vi "ResonanceAnalyzer.vi"() -> ()   [LabVIEW 2015]
uses:
  <vilib>/imath/engines/lvmath2/RunTimeEngine/Managers/WorkSpace/UID Generator.vi
  <vilib>/imath/engines/lvmath2/RunTimeEngine/RangeToken/NIMS_Range.vi
  <instcachedir>/0/NIMS_Range_D919CC09935940E88F755EC1C6F49AC1.lvgen/NIMS_Range_D919CC09935940E88F755EC1C6F49AC1_000.vi
  <vilib>/imath/engines/lvmath2/RunTimeEngine/RunTimeType/NIMS_RunTimeType_From StrictType (excl LVString).vi
  <instcachedir>/0/NIMS_RunTimeType_From StrictType (excl LVString)_EB1C38A9BC5048DA9ABDA8F781E54D21.lvgen/NIMS_RunTimeType_From StrictType (excl LVString)_EB1C38A9BC5048DA9ABDA8F781E54D21_000.vi
  <vilib>/imathl/engines/lvmath/Functions/Error Handling/Create Error.vi
  <vilib>/imath/engines/lvmath2/RunTimeEngine/LocalVariableDefStatement/MC_LocalVariableDefStatement_Display.vi
  <vilib>/imath/engines/lvmath2/RunTimeEngine/ArithmeticOperatorToken/NIMS_ArithmeticOperator_minus.vi
  <instcachedir>/0/NIMS_ArithmeticOperator_minus_8228ED1EA52B4CB8A68367813E4B0C9D.lvgen/NIMS_ArithmeticOperator_minus_8228ED1EA52B4CB8A68367813E4B0C9D_003.vi
  <vilib>/imath/engines/lvmath2/RunTimeEngine/BuiltInFunctions/randnormal/NIMS_randnormal(1,I32).vi
  <vilib>/imath/engines/lvmath2/RunTimeEngine/ErrorHandling/NIMS_Error From Error Code.vi
  <vilib>/imath/engines/lvmath2/RunTimeEngine/ArithmeticOperatorToken/NIMS_ArithmeticOperator_plus.vi
  <instcachedir>/0/NIMS_ArithmeticOperator_plus_A4F2756F5ADB4A0090E0DBD7C10701C8.lvgen/NIMS_ArithmeticOperator_plus_A4F2756F5ADB4A0090E0DBD7C10701C8_000.vi
  <vilib>/imath/engines/lvmath2/RunTimeEngine/Managers/SymbolTable/Clear UID.vi
  <vilib>/imath/engines/lvmath2/RunTimeEngine/NodeEndStatement/NIMS_NodeEndStatement_Output.vi
  <instcachedir>/0/NIMS_NodeEndStatement_Output_53EC0D466D134D7ABD903AC30B43404B.lvgen/NIMS_NodeEndStatement_Output_53EC0D466D134D7ABD903AC30B43404B_000.vi
  <instcachedir>/0/NIMS_NodeEndStatement_Output_53EC0D466D134D7ABD903AC30B43404B.lvgen/NIMS_NodeEndStatement_Output_53EC0D466D134D7ABD903AC30B43404B_005.vi
  <vilib>/imath/engines/lvmath2/RunTimeEngine/ErrorHandling/NIMS_Finalize Error.vi
  <vilib>/imath/engines/lvmath2/RunTimeEngine/Managers/SymbolTable/NIMS_WorkSpace.lvlib
panel:
  out "Resonance Curve":cluster{"all rows":dbl[], "gaus":dbl[]}[](graph)=[{"all rows"=[400.0, 405.0, 410.0, 415.0, 420.0, 425.0, 430.0, 435.0, 440.0, 445.0, 450.0, 455.0, 460.0, 465.0, 470.0, 475.0, 480.0, 485.0, 490.0, 495.0, 500.0, 505.0, 510.0, 515.0, 520.0, 525.0, 530.0, 535.0, 540.0, 545.0, 550.0, 555.0, 560.0, 565.0, 570.0, 575.0, 580.0, 585.0, 590.0, 595.0, 600.0, 605.0, 610.0, 615.0, 620.0, 625.0, 630.0, 635.0, 640.0, 645.0, 650.0, 655.0, 660.0, 665.0, 670.0, 675.0, 680.0, 685.0, 690.0, 695.0, 700.0, 705.0, 710.0, 715.0, 720.0, 725.0, 730.0, 735.0, 740.0, 745.0, 750.0, 755.0, 760.0, 765.0, 770.0, 775.0, 780.0, 785.0, 790.0, 795.0, 800.0], "gaus"=[0.11351255241604037, 0.10414222503354348, 0.14444483533821953, 0.12748302072615827, 0.14497389221892898, 0.14384673103899848, 0.13374578408031648, 0.14179280076944742, 0.17330958944267544, 0.15907169164132778, 0.16753655176934548, 0.16514207171692954, 0.17190989932736572, 0.19691614978271704, 0.20190504370869367, 0.19441310786291455, 0.2133039056485444, 0.22477415941804885, 0.23020971646198585, 0.24797121378470008, 0.2536933279412255, 0.2773465910547763, 0.301521430656102, 0.30956997750864884, 0.33249213036731134, 0.34901602097743123, 0.39769074122820985, 0.41031887916188703, 0.41035673261766525, 0.4711874530017596, 0.48766721146953573, 0.5492859462216138, 0.5898183790247801, 0.6438836611617386, 0.7018972947086338, 0.7573592265847696, 0.8210938003460564, 0.8853988418295023, 0.9371620585856762, 0.9801248705682459, 0.9925356919276602, 0.9826137332493343, 0.9416889179435013, 0.9038575366906659, 0.8387554089811039, 0.7514021523756544, 0.7110991566651323, 0.6551377055862742, 0.6094819615126883, 0.5538177650246402, 0.5319943007321655, 0.48910912426227615, 0.4664119707496909, 0.44299884166073034, 0.40749275213784797, 0.38106205184860775, 0.3556589604478616, 0.3525103630210351, 0.3440871075427643, 0.31533845119817244, 0.29976668536036305, 0.2783162631954814, 0.2906476775521945, 0.2780539999902984, 0.26105862787721157, 0.255426074204126, 0.24557287287082505, 0.23745403917037838, 0.2423146884104632, 0.23349863360954015, 0.2027924510768934, 0.2039658188408361, 0.19926647781431656, 0.19642032188296885, 0.19371971901273244, 0.1916702535490835, 0.18835962796664552, 0.17745845067880478, 0.17841560928600508, 0.171532214028235, 0.15443785512252695]}, {"all rows"=[400.0, 405.0, 410.0, 415.0, 420.0, 425.0, 430.0, 435.0, 440.0, 445.0, 450.0, 455.0, 460.0, 465.0, 470.0, 475.0, 480.0, 485.0, 490.0, 495.0, 500.0, 505.0, 510.0, 515.0, 520.0, 525.0, 530.0, 535.0, 540.0, 545.0, 550.0, 555.0, 560.0, 565.0, 570.0, 575.0, 580.0, 585.0, 590.0, 595.0, 600.0, 605.0, 610.0, 615.0, 620.0, 625.0, 630.0, 635.0, 640.0, 645.0, 650.0, 655.0, 660.0, 665.0, 670.0, 675.0, 680.0, 685.0, 690.0, 695.0, 700.0, 705.0, 710.0, 715.0, 720.0, 725.0, 730.0, 735.0, 740.0, 745.0, 750.0, 755.0, 760.0, 765.0, 770.0, 775.0, 780.0, 785.0, 790.0, 795.0, 800.0], "gaus"=[0.11892435654300736, 0.12282734325640836, 0.12692064160827352, 0.1312191490068874, 0.13573931751779073, 0.14049935888608772, 0.14551948218171426, 0.15082217013157131, 0.15643250148251903, 0.16237852831753594, 0.1686917191977432, 0.17540748141751927, 0.18256577865249124, 0.1902118639900121, 0.19839715292579332, 0.20718026658252003, 0.21662828236911227, 0.2268182377606916, 0.23783894298854777, 0.24979317016415276, 0.2628002993015277, 0.2769995145893434, 0.2925536541534718, 0.30965381719781526, 0.3285248112128024, 0.3494314541621426, 0.3726855845009083, 0.398653284759308, 0.4277611217393421, 0.46049883371853045, 0.4974132905863116, 0.5390837703827893, 0.5860602321846007, 0.6387328739972306, 0.6970835970975545, 0.7602583531668472, 0.8259306283577391, 0.889583744570278, 0.9442088756583177, 0.9813204872080571, 0.9938278398123565, 0.9794874661552115, 0.942116222283669, 0.8894089891945062, 0.8294446788572712, 0.7684099929054267, 0.71009198407197, 0.6563567849513765, 0.6078379714990343, 0.5644878254485798, 0.5259323812265361, 0.4916737817486462, 0.461195544276965, 0.4340121392138449, 0.40968870161218524, 0.38784564078411693, 0.36815616430643266, 0.3503408990520392, 0.3341617018584087, 0.3194156449035439, 0.3059295890974517, 0.29355547319307834, 0.28216631097381767, 0.271652830925331, 0.26192067362005517, 0.2528880613855749, 0.2444838622430286, 0.23664598032865905, 0.22932001551601336, 0.22245814461604568, 0.21601818494044386, 0.20996280811029483, 0.20425887787418834, 0.19887689052195087, 0.19379050040813722, 0.18897611628788566, 0.18441255675214577, 0.18008075514383087, 0.17596350603541955, 0.17204524672877594, 0.1683118683615231]}]
  out "Results":T1={"Amplitude"=0.9938486787549025, "Q"=9.964741129222524, "Center Frequency"=599.8050675226251}
  in  "?":enum32{"Simulation", "Experiment"}(tab)
  in  "Input Parameters":T2={"Q"=10.0, "End Frequency"=800.0, "df"=5.0, "Noise Level"=0.01, "Center Frequency"=600.0, "Start Frequency"=400.0}
  in  "file path (dialog if empty)":path
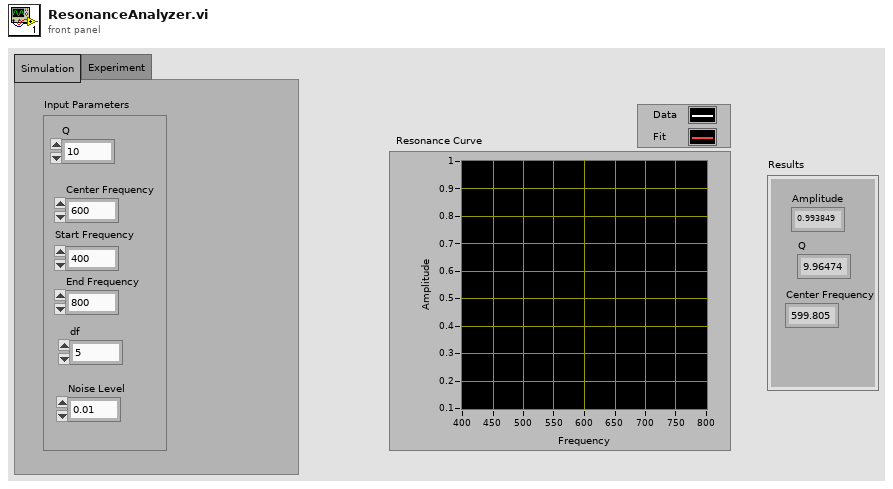
[diagram p1: front panel]
types:
  T1 = cluster{"Amplitude":dbl, "Q":dbl, "Center Frequency":dbl}
  T2 = cluster{"Q":dbl, "End Frequency":dbl, "df":dbl, "Noise Level":dbl, "Center Frequency":dbl, "Start Frequency":dbl}
  T3 = cluster{"Array[0]":dbl, "Array[1]":dbl, "Array[2]":dbl, "Array[3]":dbl, "Array[4]":dbl, "Array[5]":dbl, "Array[6]":dbl, "Array[7]":dbl, "Array[8]":dbl}
  T4 = cluster{"Array[0]":dbl, "Array[1]":dbl, "Array[2]":dbl}
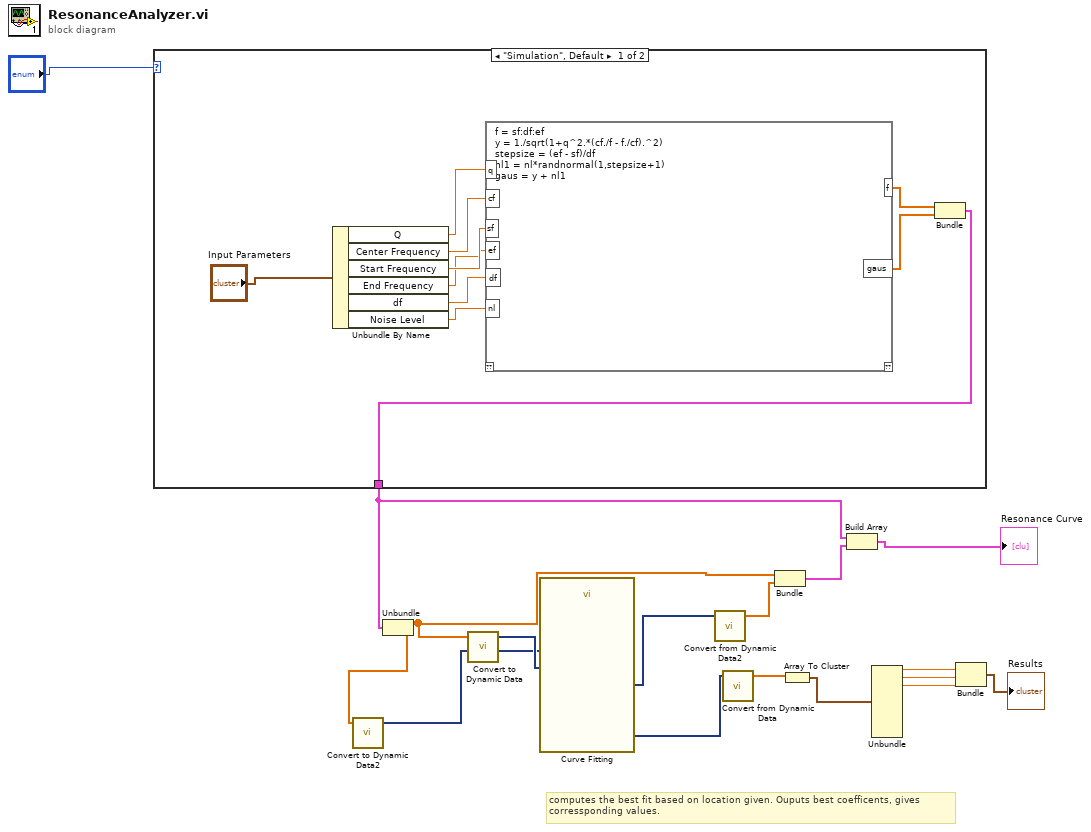
[diagram p0: block diagram]
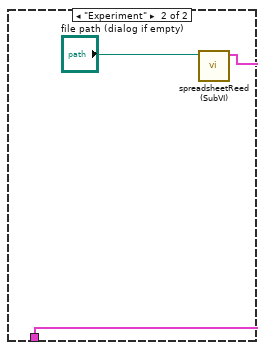
[diagram p2: hidden frame]
diagram:
  # "computes the best fit based on location given. Ouputs best coefficents, gives\ncorressponding values."
  n1 = case shown="\"Simulation\", Default" "?" {
    tunnel: [w18 w198] -> w6
    frame "Simulation", Default {
      n2 = Unbundle By Name("Input Parameters") -> ("Q"=w26:dbl, "Center Frequency"=w25:dbl, "Start Frequency"=w24:dbl, "End Frequency"=w23:dbl, "df"=w22:dbl, "Noise Level"=w21:dbl)
      n3 = mathscript code="f = sf:df:ef\ny = 1./sqrt(1+q^2.*(cf./f - f./cf).^2)\nstepsize = (ef - sf)/df\nnl1 = nl*randnormal(1,stepsize+1)\ngaus = y + nl1"("q"=w26, "cf"=w25, "sf"=w24, "ef"=w23, "df"=w22, "nl"=w21) -> ("f"=w20:dbl[], "gaus"=w19:cdb[])  [unwired: 1 in, 1 out]
      n4 = Bundle("f"=w20, "gaus"=w19) -> (w18:cluster{"f":dbl[], "gaus":cdb[]})  [unwired: 1 in]
    }
    frame "Experiment" {
      n5 = call "spreadsheetReed (SubVI).vi"("file path (dialog if empty)"="file path (dialog if empty)") -> ("Cluster"=w198:cluster{"all rows":dbl[], "all rows":dbl[]})  [unwired: 10 in]
    }
  }
  n6 = Unbundle(w6) -> ("all rows"=w10:dbl[], "gaus"=w16:cdb[])
  n7 = call "Convert to Dynamic Data2"("Array"=w16) -> ("Dynamic Data Type"=w14:dynamicdata)  [unwired: 3 in]
  n8 = call "Convert to Dynamic Data"("Array"=w10) -> ("Dynamic Data Type"=w15:dynamicdata)  [unwired: 3 in]
  n9 = call "Curve Fitting"("Locations"=w15, "Signals"=w14) -> ("best fit"=w13:dynamicdata, "non-linear coefficients"=w12:dynamicdata)  [unwired: 5 in, 3 out]
  n10 = call "Convert from Dynamic Data2"("Dynamic Data Type"=w13) -> ("Array"=w11:dbl[])  [unwired: 3 in]
  n11 = call "Convert from Dynamic Data"("Dynamic Data Type"=w12) -> ("Array"=w9:dbl[])  [unwired: 3 in]
  n12 = Bundle("all rows"=w10, "Array"=w11) -> (w7:cluster{"all rows":dbl[], "Array":dbl[]})  [unwired: 1 in]
  n13 = Array To Cluster(array=w9) -> (cluster=w8:T3)
  n14 = Build Array(w6, w7) -> (→"Resonance Curve":cluster{"all rows":dbl[], "gaus":cdb[]}[])
  n15 = Unbundle(w8) -> ("Array[0]"=w1:dbl, "Array[1]"=w2:dbl, "Array[2]"=w4:dbl)  [unwired: 6 out]
  n16 = Bundle("Array[0]"=w1, "Array[1]"=w2, "Array[2]"=w4) -> (→"Results":T4)  [unwired: 1 in]
